vi "QPD config globals.vi"() -> ()   [LabVIEW 2015]
panel:
  in  "maximum value":dbl=10.0 format="%0.2f"
  in  "minimum value":dbl=-10.0
  in  "Sampling rate (s-1)":dbl=100.0 format="%0.2f"
  in  "A-to-D channels\nfor x, y, power, supply":tag="Dev2/ai0:3"
  # "Configure QPD hardware here.  Remember to save as default."
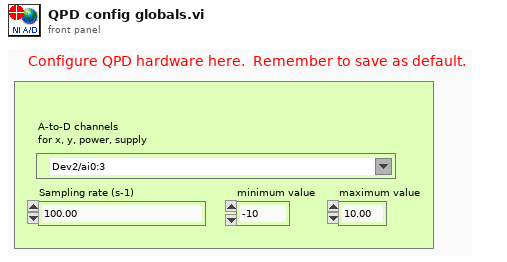
[diagram p1: front panel]
diagram:
